vi "Debug - Catch and Log.vi"(6 "Clear Error?":bool, 8 "error in (no error)":errorcluster, 11 "Debug Resources":T1) -> (0 "error out":errorcluster)   [LabVIEW 2019, in "UDP-Custom-Device Engine.lvlib"]
uses:
  UDP-Custom-Device Engine.lvlib
  Types/Engine - Debug Resources.ctl
  <vilib>/NI VeriStand/Custom Device Tools/Custom Device Utility Library/Custom Device Utility Library.lvlib
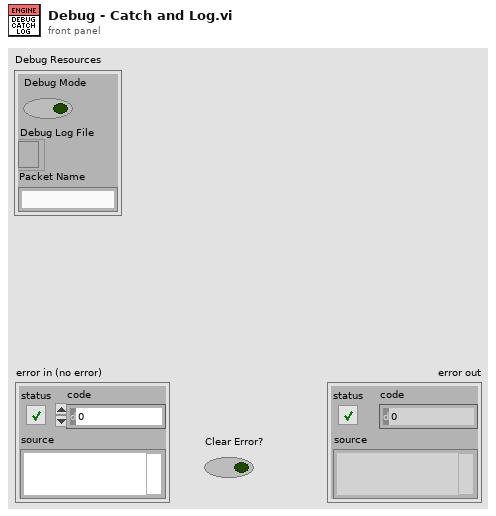
[diagram p1: front panel]
types:
  T1 = typedef "UDP-Custom-Device Engine.lvlib/Engine - Debug Resources.ctl" = cluster{"Debug Mode":bool, "Debug Log File":refnum<file>, "Packet Name":string}
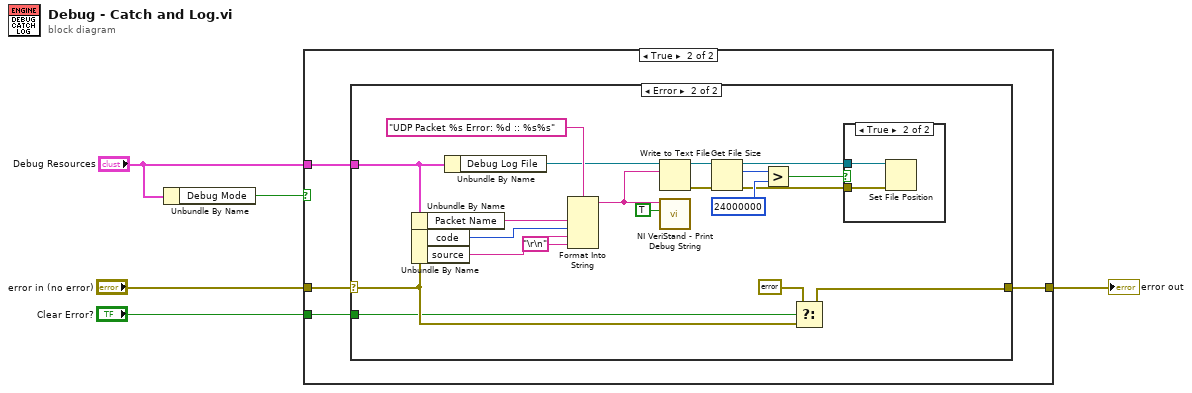
[diagram p0: block diagram]
diagram:
  n1 = Unbundle By Name("Debug Resources") -> ("Debug Mode"=w5:bool)
  n2 = case shown="True" w5 {
    tunnel: "error in (no error)" -> [w6 w10]
    tunnel: [w6 w9] -> w3
    tunnel: "Debug Resources" -> [_ w8]
    tunnel: "Clear Error?" -> [_ w7]
    frame False {
    }
    frame True {
      n3 = case shown="Error" w10 {
        selector: w10 -> [w11 w22]
        tunnel: [w11 w21] -> w9
        tunnel: w8 -> [_ w25]
        tunnel: w7 -> [_ w20]
        frame No Error {
        }
        frame Error {
          n4 = Unbundle By Name(w25) -> ("Packet Name"=w29:string)
          n5 = Unbundle By Name(w22) -> ("code"=w28:i32, "source"=w27:string)
          n6 = Unbundle By Name(w25) -> ("Debug Log File"=w24:refnum<file>)
          n7 = Format Into String(format string="UDP Packet %s Error: %d :: %s%s", w29, w28, w27, "\r\n") -> (resulting string=w23:string)  [unwired: 2 in, 1 out]
          n8 = Write to Text File(file (use dialog)=w24, text=w23) -> (refnum out=w18:refnum<file>, error out=w17:errorcluster)  [unwired: 2 in, 1 out]
          n9 = call <vilib>:"NI VeriStand - Print Debug String.vi"("Add to log file? (F)"=TRUE ("Add to log file? (T)"), "Message"=w23) -> ()  [unwired: 9 in, 1 out]
          n10 = Get File Size(file=w18, error in=w17) -> (refnum out=w12:refnum<file>, size (in bytes)=w16:i64, 0:w13:errorcluster)
          n11 = Greater?(x=w16, y=i64 24000000) -> (0:w14:bool)
          n12 = Select(t=errorcluster {"status"=FALSE, "code"=0, "source"=""}, s=w20, f=w22) -> (s? t:f=w21:errorcluster)
          n13 = case shown="True" w14 {
            tunnel: w13 -> [_ w32]
            tunnel: w12 -> [_ w33]
            frame False {
            }
            frame True {
              n14 = Set File Position(refnum=w33, error in=w32) -> ()  [unwired: 2 in, 2 out]
            }
          }
        }
      }
    }
  }
  "error out" <- w3
